vi "solar_msg Q Wait.vi"(4 "CMD_DATA Array":variant[](array[variant]), 5 "Priority (Normal)":enum8{"Normal", "Priority", "IgnoreIfExists"}(ring), 6 "CMD Array":string[](array[string]), 7 "Next EnQ (0 = Now)":timestamp, 8 "error in (no error)":errorcluster, 9 "CMD_DATA (Last)":variant, 10 "CMD (Last)":string, 11 "Queue in":refnum<queue>) -> (0 "error out":errorcluster, 1 "Enqueued?":bool, 3 "Queue out":refnum<queue>)   [LabVIEW 2018]
doc: "This waits to enqueue a message specified by the future <b>Next EnQ</b> timestamp. Rather than hardcoding a wait, this waits on a preview queue so other commands can execute before enqueuing the next message."
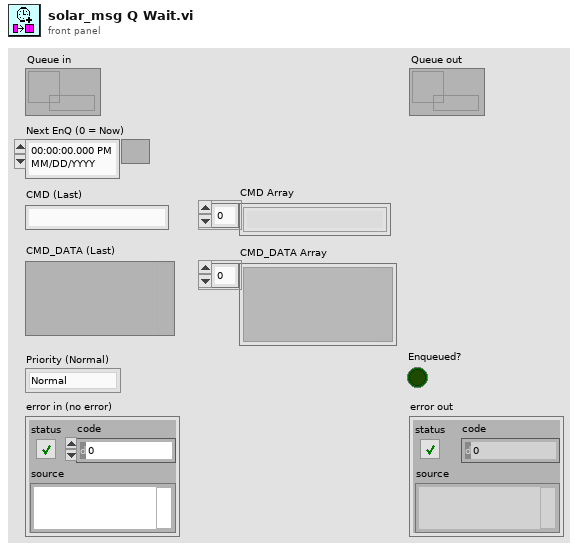
[diagram p1: front panel]
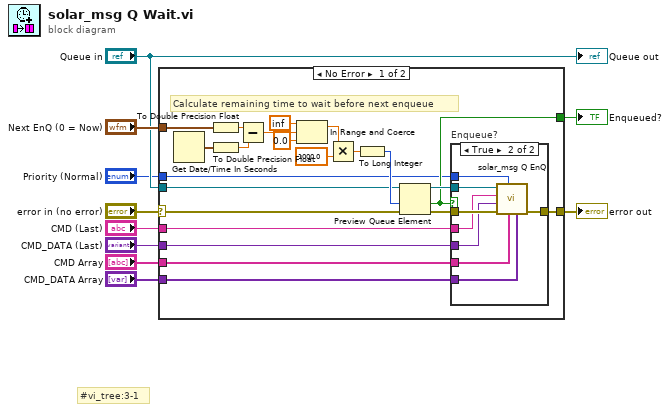
[diagram p0: block diagram]
diagram:
  # "#vi_tree:3-1"
  n1 = case shown="No Error" "error in (no error)" {
    selector: "error in (no error)" -> [w32 w42]
    tunnel: [w18 w42] -> w7
    tunnel: "Queue in" -> [w15 _]
    tunnel: "Next EnQ (0 = Now)" -> [w21 _]
    tunnel: [w16 _] -> w6
    tunnel: "CMD Array" -> [w17 _]
    tunnel: "CMD_DATA Array" -> [w14 _]
    tunnel: "Priority (Normal)" -> [w13 _]
    tunnel: "CMD (Last)" -> [w12 _]
    tunnel: "CMD_DATA (Last)" -> [w11 _]
    frame No Error {
      # "Calculate remaining time to wait before next enqueue"
      n2 = Get Date/Time In Seconds() -> (seconds since 1Jan1904=w31:timestamp)
      n3 = To Double Precision Float(number=w21) -> (double precision float=w29:dbl)
      n4 = To Double Precision Float(number=w31) -> (double precision float=w30:dbl)
      n5 = Subtract(x=w29, y=w30) -> (x-y=w28:dbl)
      n6 = In Range and Coerce(upper limit=inf ("Positive Infinity"), x=w28, lower limit=0.0) -> (coerced(x)=w25:dbl)  [unwired: 1 out]
      n7 = Multiply(x=w25, y=1000.0 ("x")) -> (x*y=w24:dbl)
      n8 = To Long Integer(number=w24) -> (32bit integer=w22:i32)
      n9 = Preview Queue Element(queue=w15, timeout in ms (-1)=w22, error in (no error)=w32) -> (queue out=w20:refnum<queue>, timed out?=w16:bool, error out=w19:errorcluster)  [unwired: 1 out]
      n10 = case "Enqueue?" shown="True" w16 {
        tunnel: w20 -> [_ w40]
        tunnel: w19 -> [w33 w41]
        tunnel: [w33 w38] -> w18
        tunnel: w17 -> [_ w36]
        tunnel: w14 -> [_ w37]
        tunnel: w13 -> [_ w39]
        tunnel: w12 -> [_ w35]
        tunnel: w11 -> [_ w34]
        frame False {
        }
        frame True {
          n11 = call "solar_msg Q EnQ.vi"("CMD_DATA Array"=w37, "CMD Array"=w36, "Priority (Normal)"=w39, "error in (no error)"=w41, "CMD_DATA (Last)"=w34, "CMD (Last)"=w35, "Queue in"=w40) -> ("error out"=w38:errorcluster)  [unwired: 2 in, 2 out]
        }
      }
    }
    frame Error {
    }
  }
  "error out" <- w7
  "Enqueued?" <- w6
  "Queue out" <- "Queue in"
